vi "MatrixMean.vi"(11 "Real Matrix":T1) -> (0 "time":i32[](array[numeric]), 1 "DevStd Assoluta":dbl[](array[numeric]), 3 "Mean":dbl[](array[numeric]))   [LabVIEW 2014]
uses:
  <vilib>/Analysis/Matrix/Datatypes/RealMatrix.ctl
  <vilib>/Analysis/NI_AALBase.lvlib
  <vilib>/Analysis/Matrix/NI_Matrix.lvlib
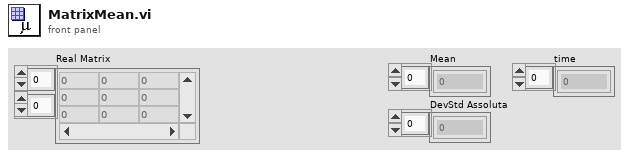
[diagram p1: front panel]
types:
  T1 = typedef "NI_Matrix.lvlib/RealMatrix.ctl" = dbl[][]
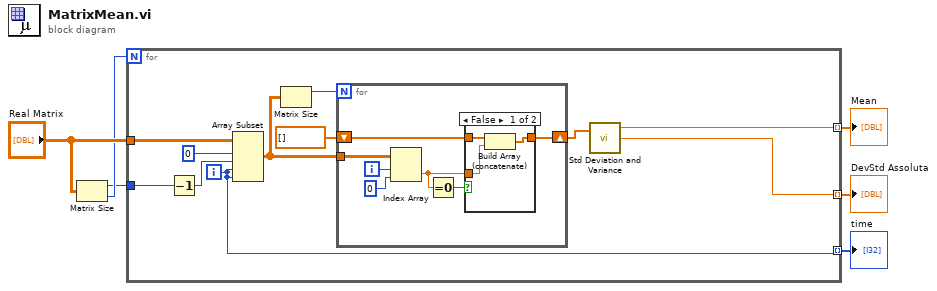
[diagram p0: block diagram]
diagram:
  n1 = Matrix Size(0:"Real Matrix") -> (1:w4:i32, 2:w5:i32)
  n2 = for {
    N: w5 -> [_]
    tunnel: "Real Matrix" -> [w17]
    tunnel: w4 -> [w15]
    tunnel: [w9] -> w3 mode=indexing
    tunnel: [w8] -> w2 mode=indexing
    tunnel: [w7] -> w1 mode=indexing
    i -> [w7]
    n3 = Decrement(x=w15) -> (x-1=w14:i32)
    n4 = Array Subset(array=w17, index (row)=0 ("row 1"), length (row)=w14, index (col)=w7, length (col)=w7) -> (w13:T1)
    n5 = Matrix Size(0:w13) -> (1:w12:i32)  [unwired: 1 out]
    n6 = for {
      N: w12 -> [_]
      tunnel: w13 -> [w22]
      shift-right: [w18] -> w10
      shift-left: dbl[] [] ("Array") -> [w21]
      i -> [w24]
      n7 = Index Array(array=w22, index (row)=w24, index (col)=0) -> (element=w20:dbl)
      n8 = Equal To 0?(x=w20) -> (x = 0?=w19:bool)
      n9 = case shown="False" w19 {
        tunnel: w21 -> [w27 w28]
        tunnel: w20 -> [w26 _]
        tunnel: [w25 w28] -> w18
        frame False {
          n10 = Build Array (concatenate)(w27, w26) -> (w25:dbl[])
        }
        frame True {
        }
      }
    }
    n11 = call <vilib>:"Std Deviation and Variance.vi"("X"=w10) -> ("mean"=w9:dbl, "standard deviation"=w8:dbl)  [unwired: 1 in, 1 out]
  }
  "Mean" <- w3
  "DevStd Assoluta" <- w2
  "time" <- w1
